vi "Send Climb Data.vi"(10 "DVR In":refnum<data-value>) -> ()   [LabVIEW 2016]
uses:
  Climb Notifier.ctl
  Climb Control Type.ctl
  Climb Globals.vi
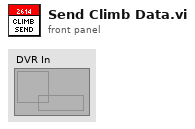
[diagram p1: front panel]
types:
  T1 = typedef "Climb Notifier.ctl" = cluster{"Up":bool, "Down":bool, "Climb Control List":T2}
  T2 = typedef "Climb Control Type.ctl" = enum16{"No Op", "Up", "Down"}
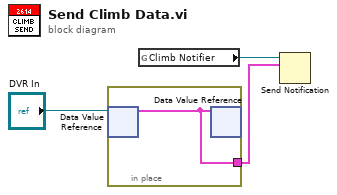
[diagram p0: block diagram]
diagram:
  n1 = in-place {
    in-place-border: [w4] -> w2
    n2 = in-place-dvr #1("DVR In") -> (w4:T1)  [unwired: 1 out]
    n3 = in-place-dvr #1(w4) -> ()  [unwired: 2 out]
  }
  n4 = global read "Climb Globals.vi" "Climb Notifier"() -> (w1:refnum<notifier>)
  n5 = Send Notification(notification=w2, notifier=w1) -> ()  [unwired: 1 in, 2 out]
